vi "DDSSequence_Ramp.vi"() -> ()   [LabVIEW 2016]
panel:
  in  "Freqeuncy (MHz)":dbl[][](array[numeric])=[[1.0, 2.0, 2.0, 1.0, 0.5, 0.0]]
  in  "Power":dbl[][](array[numeric])=[[1.0, 0.0, 0.5, 0.0, 1.0, 0.0]]
  out "Instruction String Slot 2":string="dds 0 reset\rdcp 0 spi:CFR2=0x1000080\rdcp 0 spi:STP0=0x418937\rdcp 0 wait::BNC_IN_A_RISING\rdcp 0 update:u\rdcp 0 spi:STP0=0x3FFF000000418937\rdcp 0 wait:0h:\rdcp 0 update:u\r\rdcp 0 spi:STP0=0x83126F\rdcp 0 wait:62500h:\rdcp 0 update:u\r\rdcp 0 spi:STP0=0x3FFF00000083126F\rdcp 0 wait:31250h:\rdcp 0 update:u\r\rdcp 0 spi:STP0=0x418937\rdcp 0 wait:62500h:\rdcp 0 update:u\r\rdcp 0 spi:DRL=0xFFFC000000000000\rdcp 0 spi:DRSS=0x28F5C29028F5C29\rdcp 0 spi:DRR=0x1F401F4\rdcp 0 spi:CFR2=0x280080\rdcp 0 wait:62500h:\rdcp 0 update:u+d\rdcp 0 wait:125000h:\rdcp 0 update:-d\rdcp 0 spi:CFR2=0x1200080\rdcp 0 spi:STP0=0x418937\rdcp 0 wait:62500h:\rdcp 0 update:u\rdcp 0 start\rdds 1 reset\rdcp 1 spi:CFR2=0x1000080\rdcp 1 spi:STP0=0x418937\rdcp 1 wait::BNC_IN_A_RISING\rdcp 1 update:u\rdcp 1 spi:STP0=0x3FFF000000418937\rdcp 1 wait:0h:\rdcp 1 update:u\r\rdcp 1 spi:STP0=0x83126F\rdcp 1 wait:62500h:\rdcp 1 update:u\r\rdcp 1 spi:STP0=0x200000000083126F\rdcp 1 wait:31250h:\rdcp 1 update:u\r\rdcp 1 spi:STP0=0x418937\rdcp 1 wait:62500h:\rdcp 1 update:u\r\rdcp 1 spi:DRL=0xFFFC000000000000\rdcp 1 spi:DRSS=0x28F5C29028F5C29\rdcp 1 spi:DRR=0x1F401F4\rdcp 1 spi:CFR2=0x280080\rdcp 1 wait:62500h:\rdcp 1 update:u+d\rdcp 1 wait:125000h:\rdcp 1 update:-d\rdcp 1 spi:CFR2=0x1200080\rdcp 1 spi:STP0=0x418937\rdcp 1 wait:62500h:\rdcp 1 update:u\rdcp 1 start\r\r"
  in  "Freqeuncy (MHz)":dbl[][](array[numeric])=[[1.0, 2.0, 2.0, 1.0, 0.5, 0.0]]
  in  "Power":dbl[][](array[numeric])=[[1.0, 0.0, 1.0, 0.0, 1.0, 0.0]]
  out "return count 2":u32
  out "error out 2":errorcluster={"status"=TRUE, "code"=-1073807343, "source"="Property Node (arg 1) in VISA Configure Serial Port (Instr).vi->FlexDDS-NG_USB_VISA_Open.vi->DDSSequence.vi"}
  out "read buffer 2":string
  in  "Freqeuncy (MHz)":dbl[][](array[numeric])=[[1.0, 2.0, 2.0, 1.0, 0.5, 0.0]]
  in  "Power":dbl[][](array[numeric])=[[1.0, 0.0, 0.5, 0.0, 1.0, 0.0]]
  out "Instruction String Slot 1":string="dds 0 reset\rdcp 0 spi:CFR2=0x1000080\rdcp 0 spi:STP0=0x418937\rdcp 0 wait::BNC_IN_A_RISING\rdcp 0 update:u\rdcp 0 spi:STP0=0x3FFF000000418937\rdcp 0 wait:0h:\rdcp 0 update:u\r\rdcp 0 spi:STP0=0x83126F\rdcp 0 wait:62500h:\rdcp 0 update:u\r\rdcp 0 spi:STP0=0x3FFF00000083126F\rdcp 0 wait:31250h:\rdcp 0 update:u\r\rdcp 0 spi:STP0=0x418937\rdcp 0 wait:62500h:\rdcp 0 update:u\r\rdcp 0 spi:DRL=0xFFFC000000000000\rdcp 0 spi:DRSS=0x28F5C29028F5C29\rdcp 0 spi:DRR=0x1F401F4\rdcp 0 spi:CFR2=0x280080\rdcp 0 wait:62500h:\rdcp 0 update:u+d\rdcp 0 wait:125000h:\rdcp 0 update:-d\rdcp 0 spi:CFR2=0x1200080\rdcp 0 spi:STP0=0x418937\rdcp 0 wait:62500h:\rdcp 0 update:u\rdcp 0 start\rdds 1 reset\rdcp 1 spi:CFR2=0x1000080\rdcp 1 spi:STP0=0x418937\rdcp 1 wait::BNC_IN_A_RISING\rdcp 1 update:u\rdcp 1 spi:STP0=0x3FFF000000418937\rdcp 1 wait:0h:\rdcp 1 update:u\r\rdcp 1 spi:STP0=0x83126F\rdcp 1 wait:62500h:\rdcp 1 update:u\r\rdcp 1 spi:STP0=0x200000000083126F\rdcp 1 wait:31250h:\rdcp 1 update:u\r\rdcp 1 spi:STP0=0x418937\rdcp 1 wait:62500h:\rdcp 1 update:u\r\rdcp 1 spi:DRL=0xFFFC000000000000\rdcp 1 spi:DRSS=0x28F5C29028F5C29\rdcp 1 spi:DRR=0x1F401F4\rdcp 1 spi:CFR2=0x280080\rdcp 1 wait:62500h:\rdcp 1 update:u+d\rdcp 1 wait:125000h:\rdcp 1 update:-d\rdcp 1 spi:CFR2=0x1200080\rdcp 1 spi:STP0=0x418937\rdcp 1 wait:62500h:\rdcp 1 update:u\rdcp 1 start\r\r"
  in  "No of  active time blocks":dbl=4.0
  in  "Freqeuncy (MHz)":dbl[][](array[numeric])=[[1.0, 2.0, 2.0, 1.0, 0.5, 0.0]]
  in  "Duration (ms)":dbl[][](array[numeric])=[[0.5, 0.25, 0.5, 1.0, 2.0, 1.0]]
  in  "Power":dbl[][](array[numeric])=[[1.0, 0.0, 1.0, 0.0, 1.0, 0.0]]
  out "return count":u32=1275
  out "error out":errorcluster={"status"=TRUE, "code"=-1073807339, "source"="VISA Read in DDSSequence.vi"}
  out "read buffer":string
  # "DDS 0"
  # "DDS 1"
  # "DDS 3"
  # "DDS 4"
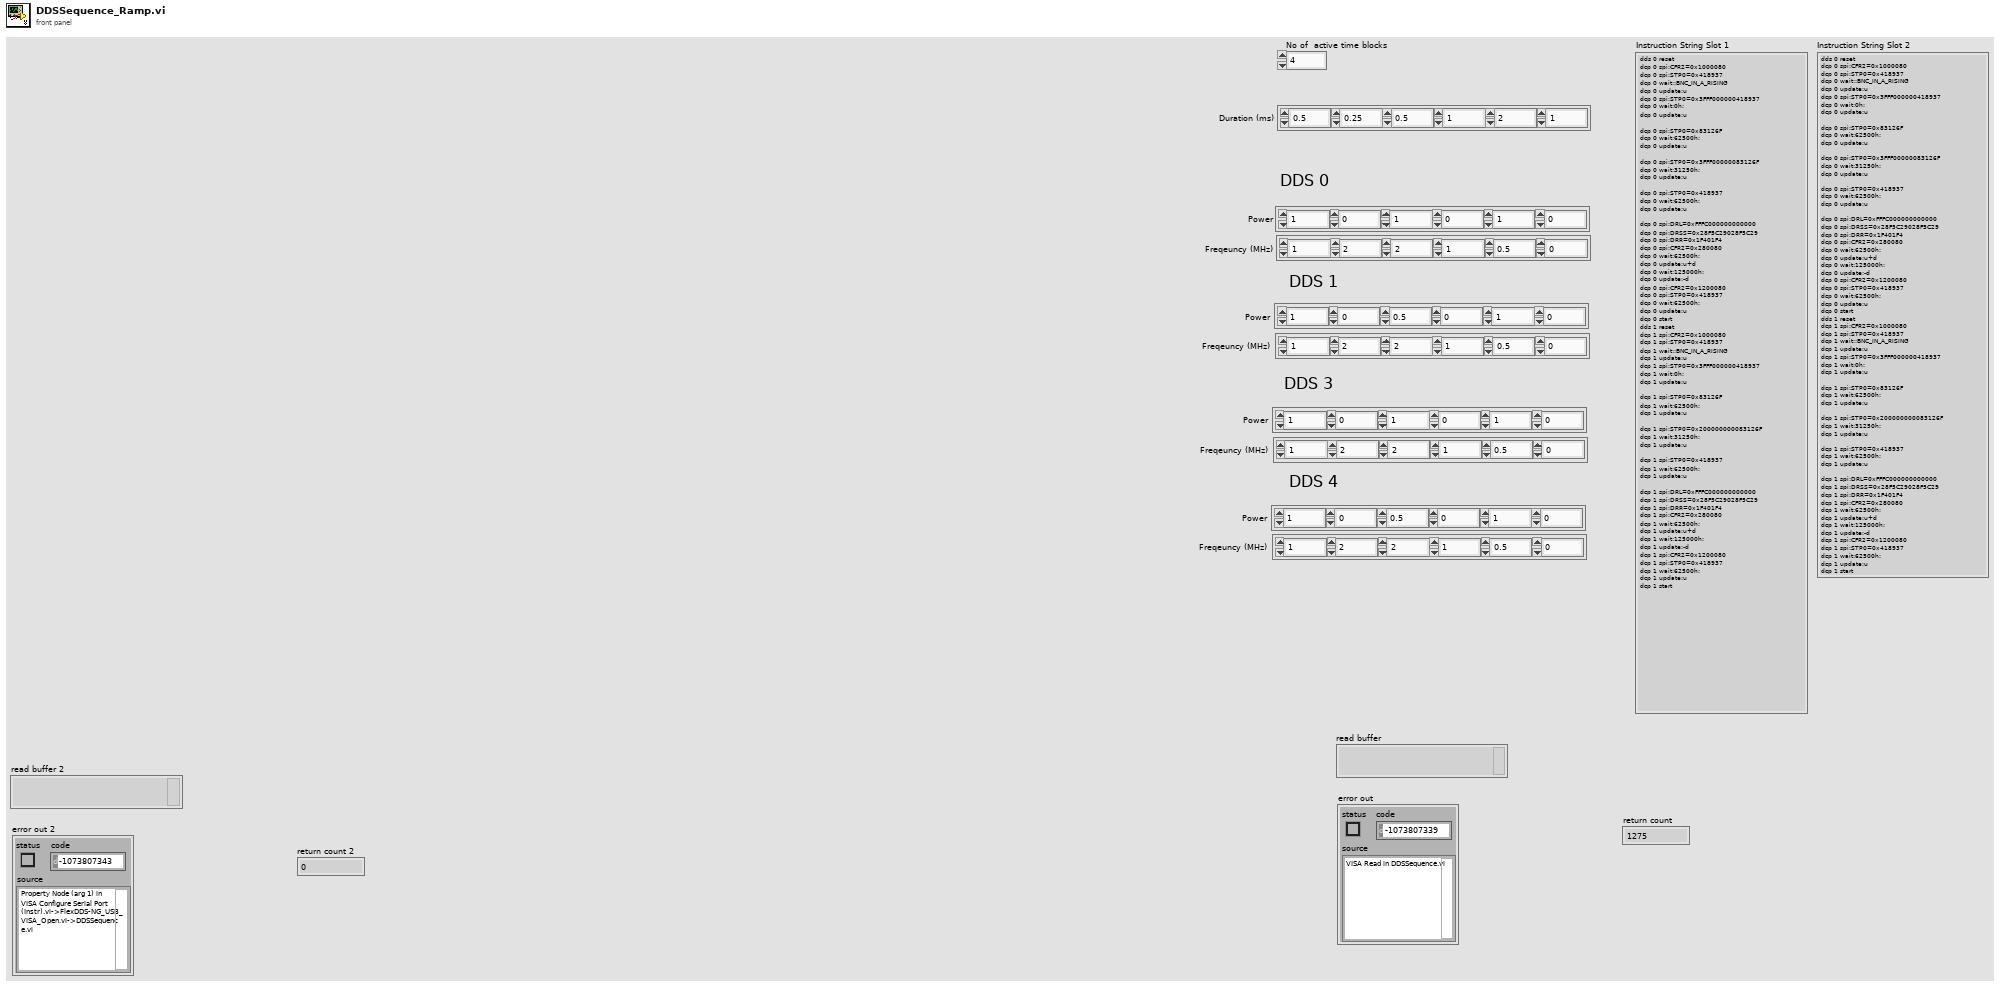
[diagram p1: front panel]
types:
  T1 = enum32{"Channel 0", "Channel 1", "Both channels"}
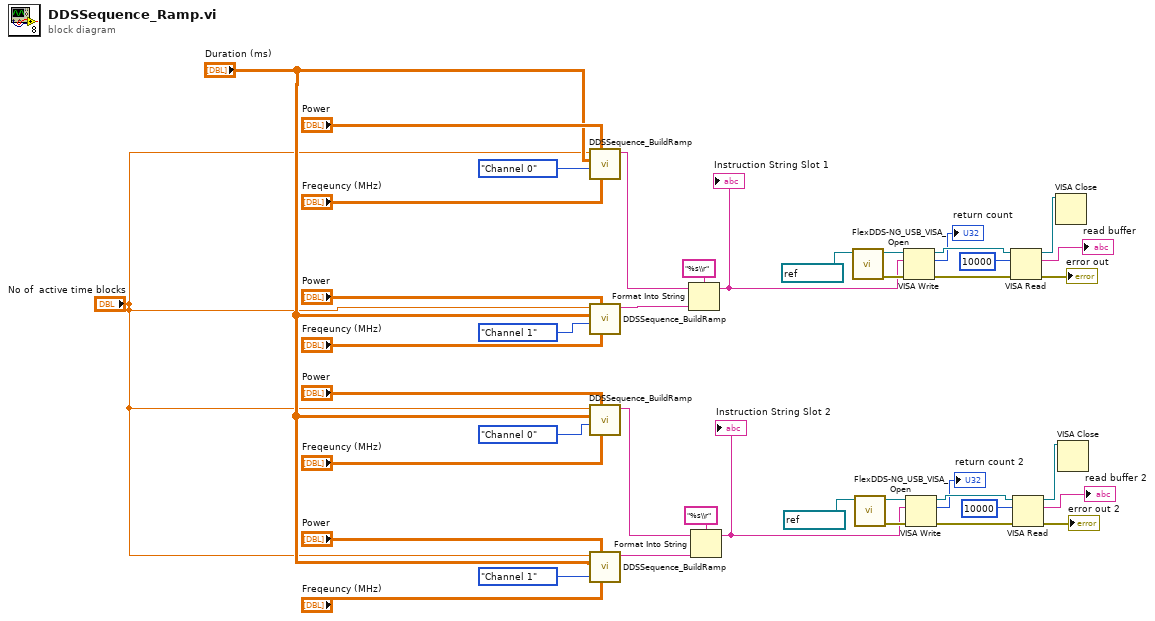
[diagram p0: block diagram]
diagram:
  n1 = call "DDSSequence_BuildRamp.vi"("Freqeuncy (MHz)"="Freqeuncy (MHz)", "Power"="Power", "Channels"=T1."Channel 0", "Duration (ms)"="Duration (ms)", "No of  active time blocks"="No of  active time blocks") -> ("appended instruction string"=w6:string)  [unwired: 6 in]
  n2 = call "DDSSequence_BuildRamp.vi"("Freqeuncy (MHz)"="Freqeuncy (MHz)", "Power"="Power", "Channels"=T1."Channel 1", "Duration (ms)"="Duration (ms)", "No of  active time blocks"="No of  active time blocks") -> ("appended instruction string"=w10:string)  [unwired: 6 in]
  n3 = call "DDSSequence_BuildRamp.vi"("Freqeuncy (MHz)"="Freqeuncy (MHz)", "Power"="Power", "Channels"=T1."Channel 0", "Duration (ms)"="Duration (ms)", "No of  active time blocks"="No of  active time blocks") -> ("appended instruction string"=w14:string)  [unwired: 6 in]
  n4 = call "DDSSequence_BuildRamp.vi"("Freqeuncy (MHz)"="Freqeuncy (MHz)", "Power"="Power", "Channels"=T1."Channel 1", "Duration (ms)"="Duration (ms)", "No of  active time blocks"="No of  active time blocks") -> ("appended instruction string"=w2:string)  [unwired: 6 in]
  n5 = Format Into String(format string="%s\\r", initial string=w6, w10) -> (resulting string=w31:string)  [unwired: 1 in, 1 out]
  "Instruction String Slot 1" <- w31
  n6 = Format Into String(format string="%s\\r", initial string=w14, w2) -> (resulting string=w16:string)  [unwired: 1 in, 1 out]
  "Instruction String Slot 2" <- w16
  n7 = call "FlexDDS-NG_USB_VISA_Open.vi"("FlexDDS-NG USB VISA resource name (COM)"=refnum<visa-resource-name> "COM7") -> ("error out"=w34:errorcluster, "FlexDDS-NG USB VISA resource name out"=w35:refnum<visa-resource-name>)  [unwired: 9 in]
  n8 = call "FlexDDS-NG_USB_VISA_Open.vi"("FlexDDS-NG USB VISA resource name (COM)"=refnum<visa-resource-name> "COM8") -> ("error out"=w22:errorcluster, "FlexDDS-NG USB VISA resource name out"=w23:refnum<visa-resource-name>)  [unwired: 9 in]
  n9 = VISA Write(VISA resource name=w35, write buffer=w31, error in (no error)=w34) -> (VISA resource name out=w39:refnum<visa-resource-name>, return count=→"return count":u32, error out=w37:errorcluster)
  n10 = VISA Write(VISA resource name=w23, write buffer=w16, error in (no error)=w22) -> (VISA resource name out=w27:refnum<visa-resource-name>, return count=→"return count 2":u32, error out=w25:errorcluster)
  n11 = VISA Read(VISA resource name=w39, byte count=u32 10000, error in (no error)=w37) -> (VISA resource name out=w42:refnum<visa-resource-name>, read buffer=→"read buffer":string, error out=→"error out":errorcluster)  [unwired: 1 out]
  n12 = VISA Read(VISA resource name=w27, byte count=u32 10000, error in (no error)=w25) -> (VISA resource name out=w30:refnum<visa-resource-name>, read buffer=→"read buffer 2":string, error out=→"error out 2":errorcluster)  [unwired: 1 out]
  n13 = VISA Close(VISA resource name=w42) -> ()  [unwired: 1 in, 1 out]
  n14 = VISA Close(VISA resource name=w30) -> ()  [unwired: 1 in, 1 out]
